vi "获取返回参数有效数据.vi"(9 "帧首数据":string="+RECW0", 10 "输入字符串输入":string) -> (2 "是否有效数据":bool, 3 "输入字符串输出":string)   [LabVIEW 2015]
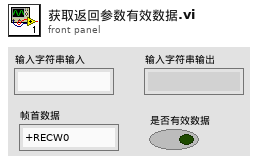
[diagram p1: front panel]
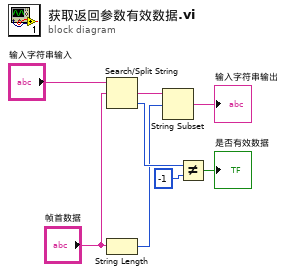
[diagram p0: block diagram]
diagram:
  n1 = Search/Split String(string="输入字符串输入", search string/char (-)="帧首数据") -> (match + rest of string=w3:string, offset of match=w6:i32)  [unwired: 1 in, 1 out]
  n2 = String Length(string="帧首数据") -> (length=w2:i32)
  n3 = String Subset(string=w3, offset (0)=w2) -> (substring=→"输入字符串输出":string)  [unwired: 1 in]
  n4 = Not Equal?(x=w6, y=-1) -> (x != y?=→"是否有效数据":bool)
